vi "Hannah's Simulator.vi"() -> ()   [LabVIEW 2024]
uses:
  <vilib>/Analysis/Matrix/Datatypes/RealMatrix.ctl
  <vilib>/Analysis/baseanly.llb/Real A x B.vi
  <vilib>/Analysis/Matrix/NI_Matrix.lvlib
  <vilib>/Analysis/NI_AALBase.lvlib
panel:
  in  "Adjust the Length!":dbl[](array[slide]) scale=0.0..2.0
  in  "Enter # of Arms:":i32=4
  in  "Adjust the Angle!":dbl[](array[slide]) scale=-90.0..90.0
  out "Hannah's Simulator":refnum<vi>(3d-picture)
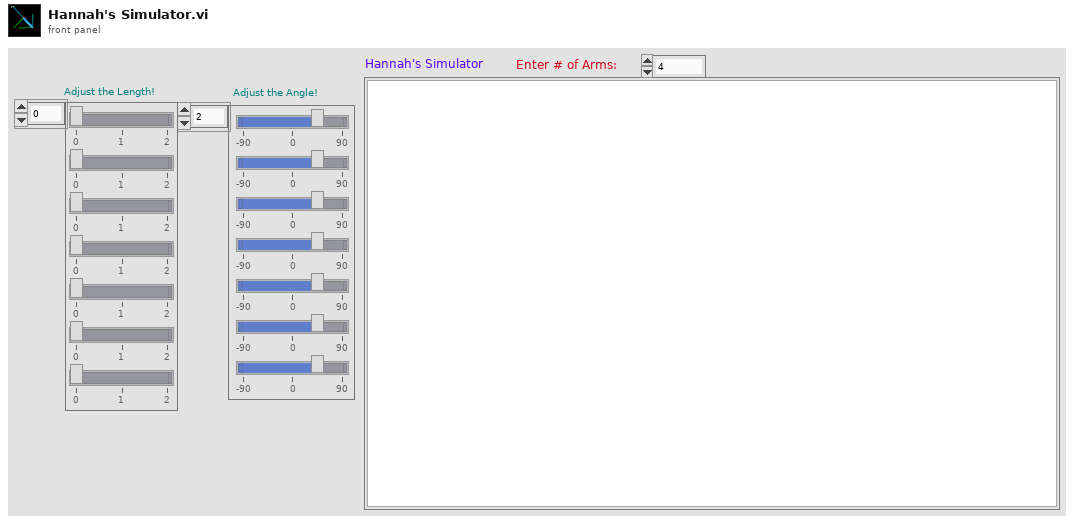
[diagram p1: front panel]
types:
  T1 = typedef "NI_Matrix.lvlib/RealMatrix.ctl" = dbl[][]
  T2 = cluster{"Line width":sgl, "Line Color":u32, "Axes?":bool}
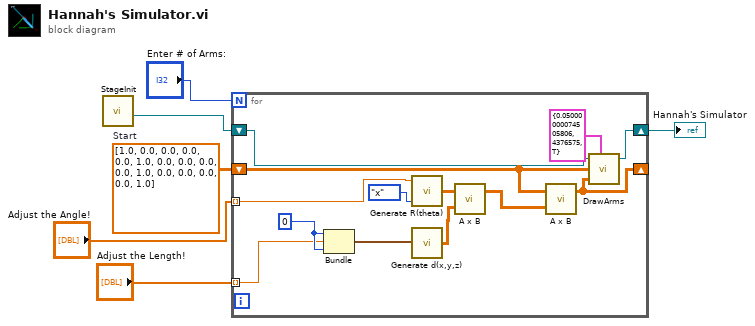
[diagram p0: block diagram]
diagram:
  w5 = T1 [[1.0, 0.0, 0.0, 0.0], [0.0, 1.0, 0.0, 0.0], [0.0, 0.0, 1.0, 0.0], [0.0, 0.0, 0.0, 1.0]]  # Start
  n1 = call <userlib>:"StageInit.vi"() -> ("Stage out"=w6:refnum<vi>)  [unwired: 4 in, 1 out]
  n2 = for {
    N: "Enter # of Arms:" -> [_]
    shift-right: [w15] -> _
    shift-left: w5 -> [w8]
    shift-right: [w13] -> w4
    shift-left: w6 -> [w16]
    tunnel: "Adjust the Angle!" -> [w10] mode=indexing
    tunnel: "Adjust the Length!" -> [w9] mode=indexing
    w12 = 0
    n3 = Bundle(w12, "Length"=w9, w12) -> (w11:cluster{i32, "Length":dbl, i32})  [unwired: 1 in]
    n4 = call <userlib>:"Generate R(theta).vi"("Axis"=enum16{"x", "y", "z"}."x", "Angle (degrees)"=w10) -> ("Transformation Matrix"=w17:T1)  [unwired: 1 in]
    n5 = call <userlib>:"Generate d(x,y,z).vi"("Translation"=w11) -> ("Transformation Matrix"=w18:T1)  [unwired: 2 in]
    n6 = call-poly <vilib>:"A x B.vi"("B"=w18, "A"=w17) -> ("A x B"=w7:T1)  [unwired: 1 out]
    n7 = call-poly <vilib>:"A x B.vi"("B"=w7, "A"=w8) -> ("A x B"=w15:T1)  [unwired: 1 out]
    n8 = call <userlib>:"DrawArms.vi"("Stage in"=w16, "Params"=T2 {"Line width"=0.05, "Line Color"=4376575, "Axes?"=TRUE}, "Start"=w8, "End"=w15) -> ("Stage out"=w13:refnum<vi>)  [unwired: 2 in, 1 out]
  }
  "Hannah's Simulator" <- w4
